vi "Configure Stream.vi"(0 "Register Bus":T1, 1 "scope":string(combo)="rx", 5 "host FIFO depth":u32=1000000 format="%.0p", 7 "number of samples is finite":bool caption="Number of Samples is Finite", 9 "number of samples":u32=8192 caption="Number of Samples", 11 "error in":errorcluster) -> (4 "Register Bus (out)":T1, 15 "error out":errorcluster)   [LabVIEW 2017]
doc: "Configure the stream. This includes configuring the DMA FIFO and the rx/tx stream size (in samples).\n\n<B>Input Parameters</B>\n\n<B>Register Bus</B> The Register Bus object created by the ni579x Open VI and used as the session handle for the NI-579x Configuration Design Library.\n\n<B>scope</B> is the channel to configure the stream for. The options are \"rx\" and \"tx\".\n\n<B>host FIFO depth</B> is the number of samples of buffering to request on the host. This value is optional and defaults to eight times the 'number of samples'.\n\n<B>number of samples is finite</B> is used to flag whether this will be a continuous or finite acquisition/generation.\n\n<B>number of samples</B> is the number of samples to acquire/generate.\n\n<B>error in</B> describes error conditions that occur before this node runs. This input provides standard 'error in' functionality.\n\n<B>Output Parameters</B>\n\n<B>Register Bus (out)</B> The Register Bus object created by the ni579x Open VI and used as the session handle for the NI-579x Configuration Design Library.\n\n<B>error out</B> contains error information. This output provides standard 'error out' functionality."
uses:
  <instrlib>/_niInstr/Register Bus/v0/Host/Public/Register Bus Session.ctl
  <instrlib>/_niInstr/Register Bus/v0/Host/Private/Session Data.ctl
  Tx FPGA VI Reference.ctl
  Rx FPGA VI Reference.ctl
  <vilib>/Utility/error.llb/Error Cluster From Error Code.vi
  <vilib>/rvi/errors/niLvFpgaAdjustHostInterfaceError.vi
  <vilib>/rvi/interface/common/niFpgaWaitOnOcc.vi
  <vilib>/rvi/interface/nirviReadWriteControl/nirviReadWriteControl.xnode
  <vilib>/rvi/interface/nirviMethod/nirviMethod.xnode
  <vilib>/ErrorRing/Error Ring.xnode
  <vilib>/rvi/errors/niLvFpgaMergeErrorWithErrorCode.vi
  <vilib>/rvi/interface/Simulation/niFpgaSimulationCallBeginRW.vi
  NiFpgaLv.dll
  <vilib>/FPGAPlugInAG/Dynamic/niLvFpga_StartFifo_Dynamic.vi
  <vilib>/FPGAPlugInAG/Dynamic/niLvFpga_StopFifo_Dynamic.vi
  <vilib>/FPGAPlugInAG/Dynamic/niLvFpga_ConfigureFifo_Dynamic.vi
  <instrlib>/_niInstr/Register Bus/v0/Host/niInstr Register Bus v0 Host.lvlib
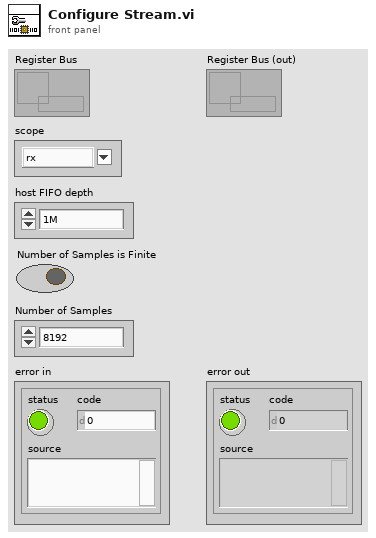
[diagram p1: front panel]
types:
  T1 = typedef "niInstr Register Bus v0 Host.lvlib/Register Bus Session.ctl" = refnum<queue>
  T2 = typedef "Tx FPGA VI Reference.ctl" = refnum<k20>
  T3 = typedef "Rx FPGA VI Reference.ctl" = refnum<k20>
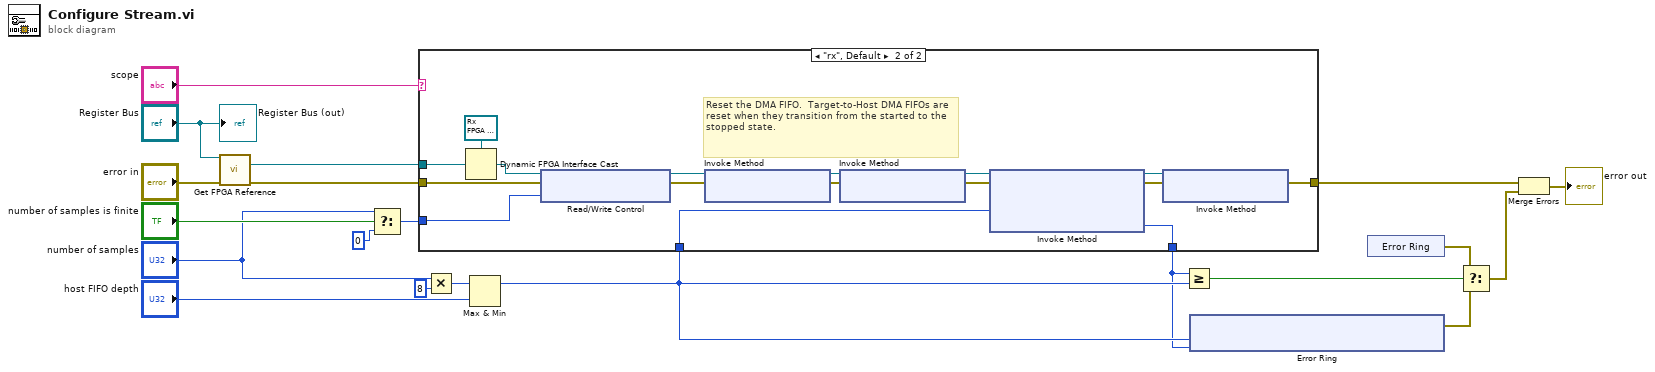
[diagram p0: block diagram]
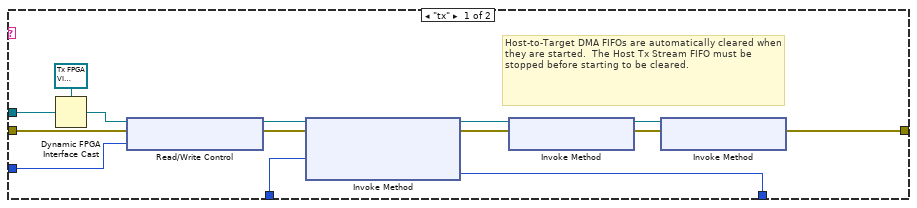
[diagram p2: hidden frame]
diagram:
  n1 = call <instrlib>:"Get FPGA Reference.vi"("session in"="Register Bus", "error in"="error in") -> ("fpga ref"=w18:refnum<k20>, "error out"=w14:errorcluster)  [unwired: 11 in, 1 out]
  n2 = Select(t="number of samples", s="number of samples is finite", f=u32 0) -> (s? t:f=w9:u32)
  n3 = Multiply(x="number of samples", y=u32 8 ("x")) -> (x*y=w16:u32)
  n4 = Max & Min(x=w16, y="host FIFO depth") -> (max(x,y)=w2:u32)  [unwired: 1 out]
  n5 = case shown="\"rx\", Default" "scope" {
    tunnel: w18 -> [w25 w50]
    tunnel: w2 -> [w23 w39]
    tunnel: [w33 w46] -> w5
    tunnel: w14 -> [w24 w44]
    tunnel: w9 -> [w22 w38]
    tunnel: [w21 w35] -> w1
    frame "tx" {
      # "Host-to-Target DMA FIFOs are automatically cleared when they are started.  The Host Tx Stream FIFO must be stopped before starting to be cleared."
      n6 = Dynamic FPGA Interface Cast(Session In=T2 refnum ("FPGA VI Reference Out"), Type=w25) -> (Session Out=w32:T2)
      n7 = xnode "Read/Write Control"("FPGA VI Reference In"=w32, "error in"=w24, "tx.samples to generate"=w22) -> ("FPGA VI Reference Out"=w30:T2, "error out"=w31:errorcluster)
      n8 = xnode "Invoke Method"("FPGA VI Reference In"=w30, "error in"=w31, "Requested Depth"=w23) -> ("FPGA VI Reference Out"=w28:T2, "error out"=w29:errorcluster, "Actual Depth"=w21:u32)
      n9 = xnode "Invoke Method"("FPGA VI Reference In"=w28, "error in"=w29) -> ("FPGA VI Reference Out"=w26:T2, "error out"=w27:errorcluster)
      n10 = xnode "Invoke Method"("FPGA VI Reference In"=w26, "error in"=w27) -> ("error out"=w33:errorcluster)  [unwired: 1 out]
    }
    frame "rx", Default {
      # "Reset the DMA FIFO.  Target-to-Host DMA FIFOs are reset when they transition from the started to the stopped state."
      n11 = Dynamic FPGA Interface Cast(Session In=T3 refnum ("Type"), Type=w50) -> (Session Out=w45:T3)
      n12 = xnode "Read/Write Control"("FPGA VI Reference In"=w45, "error in"=w44, "rx.samples to acquire"=w38) -> ("FPGA VI Reference Out"=w36:T3, "error out"=w37:errorcluster)
      n13 = xnode "Invoke Method"("FPGA VI Reference In"=w36, "error in"=w37) -> ("FPGA VI Reference Out"=w42:T3, "error out"=w43:errorcluster)
      n14 = xnode "Invoke Method"("FPGA VI Reference In"=w42, "error in"=w43) -> ("FPGA VI Reference Out"=w41:T3, "error out"=w40:errorcluster)
      n15 = xnode "Invoke Method"("FPGA VI Reference In"=w41, "error in"=w40, "Requested Depth"=w39) -> ("FPGA VI Reference Out"=w48:T3, "error out"=w47:errorcluster, "Actual Depth"=w35:u32)
      n16 = xnode "Invoke Method"("FPGA VI Reference In"=w48, "error in"=w47) -> ("error out"=w46:errorcluster)  [unwired: 1 out]
    }
  }
  n17 = Greater Or Equal?(x=w1, y=w2) -> (x >= y?=w3:bool)
  n18 = xnode ("Error Ring")("parameter 0"=w2, "parameter 1"=w1) -> ("error out"=w7:errorcluster)
  n19 = xnode ("Error Ring")() -> ("error out"=w6:errorcluster)
  n20 = Select(t=w6, s=w3, f=w7) -> (s? t:f=w8:errorcluster)
  n21 = Merge Errors(w5, w8) -> (→"error out":errorcluster)
  "Register Bus (out)" <- "Register Bus"
